vi "Create DiffIO Command.vi"(8 "error in (no error)":errorcluster, 11 "Section Ptr":T5 format="%.0x") -> (0 "error out":errorcluster, 3 "Parent Ref out":T5 format="%.0x")   [LabVIEW 2016, in "DCM System Explorer.lvlib"]
uses:
  DCM System Explorer.lvlib
  <vilib>/NI Veristand/Custom Device API/Custom Device Item Ref.ctl
  <vilib>/Powertrain Controls/Device Drivers/DCM/Diff IO/RT/Setup.ctl
  <vilib>/Powertrain Controls/Device Drivers/DCM/Diff IO/FPGA/Mode.ctl
  <vilib>/Powertrain Controls/Device Drivers/DCM/Diff IO/RT/Angle Control.ctl
  <vilib>/Powertrain Controls/Device Drivers/DCM/Diff IO/RT/Results.ctl
  <vilib>/NI Veristand/Custom Device API/Custom Device Channel Type.ctl
  Shared/DCM Constants and GUIDs.vi
  Shared/DCM Properties.vi
  <vilib>/NI VeriStand/Custom Device API/Custom Device API.lvlib
  DCM Shared.lvlib
  <vilib>/Powertrain Controls/Device Drivers/DCM/Diff IO/RT/DCM - RT - Diff IO.lvlib
  <vilib>/Powertrain Controls/Device Drivers/DCM/Diff IO/FPGA/DCM - FPGA - Diff IO.lvlib
panel:
  in  "Results":T1[](array[typedef]) {"Duty Cycle [%]" format="%#_3g"; "Frequency [Hz]" format="%#_3p"}
  in  "Setup":T2[](array[typedef])=[{"Mode"=enum."Off", "Capture Start [DBTDC]"=0.0, "Capture End [DBTDC]"=0.0, "Invert"=FALSE, "Frequency [Hz]"=0.0, "Duty Cycle [%]"=0.0, "TDC Offset [CAD]"=0.0, "Window Start [DBTDC]"=0.0, "Window End [DBTDC]"=0.0, "Angles"=[{"Enable"=FALSE, "Location [DBTDC]"=0.0, "Duration [s]"=0.0}, {"Enable"=FALSE, "Location [DBTDC]"=0.0, "Duration [s]"=0.0}, {"Enable"=FALSE, "Location [DBTDC]"=0.0, "Duration [s]"=0.0}, {"Enable"=FALSE, "Location [DBTDC]"=0.0, "Duration [s]"=0.0}], "Skip Fire"=FALSE, "Skip Fire Index"=0}, {"Mode"=enum."Off", "Capture Start [DBTDC]"=0.0, "Capture End [DBTDC]"=0.0, "Invert"=FALSE, "Frequency [Hz]"=0.0, "Duty Cycle [%]"=0.0, "TDC Offset [CAD]"=0.0, "Window Start [DBTDC]"=0.0, "Window End [DBTDC]"=0.0, "Angles"=[{"Enable"=FALSE, "Location [DBTDC]"=0.0, "Duration [s]"=0.0}, {"Enable"=FALSE, "Location [DBTDC]"=0.0, "Duration [s]"=0.0}, {"Enable"=FALSE, "Location [DBTDC]"=0.0, "Duration [s]"=0.0}, {"Enable"=FALSE, "Location [DBTDC]"=0.0, "Duration [s]"=0.0}], "Skip Fire"=FALSE, "Skip Fire Index"=0}, {"Mode"=enum."Off", "Capture Start [DBTDC]"=0.0, "Capture End [DBTDC]"=0.0, "Invert"=FALSE, "Frequency [Hz]"=0.0, "Duty Cycle [%]"=0.0, "TDC Offset [CAD]"=0.0, "Window Start [DBTDC]"=0.0, "Window End [DBTDC]"=0.0, "Angles"=[{"Enable"=FALSE, "Location [DBTDC]"=0.0, "Duration [s]"=0.0}, {"Enable"=FALSE, "Location [DBTDC]"=0.0, "Duration [s]"=0.0}, {"Enable"=FALSE, "Location [DBTDC]"=0.0, "Duration [s]"=0.0}, {"Enable"=FALSE, "Location [DBTDC]"=0.0, "Duration [s]"=0.0}], "Skip Fire"=FALSE, "Skip Fire Index"=0}, {"Mode"=enum."Off", "Capture Start [DBTDC]"=0.0, "Capture End [DBTDC]"=0.0, "Invert"=FALSE, "Frequency [Hz]"=0.0, "Duty Cycle [%]"=0.0, "TDC Offset [CAD]"=0.0, "Window Start [DBTDC]"=0.0, "Window End [DBTDC]"=0.0, "Angles"=[{"Enable"=FALSE, "Location [DBTDC]"=0.0, "Duration [s]"=0.0}, {"Enable"=FALSE, "Location [DBTDC]"=0.0, "Duration [s]"=0.0}, {"Enable"=FALSE, "Location [DBTDC]"=0.0, "Duration [s]"=0.0}, {"Enable"=FALSE, "Location [DBTDC]"=0.0, "Duration [s]"=0.0}], "Skip Fire"=FALSE, "Skip Fire Index"=0}, {"Mode"=enum."Off", "Capture Start [DBTDC]"=0.0, "Capture End [DBTDC]"=0.0, "Invert"=FALSE, "Frequency [Hz]"=0.0, "Duty Cycle [%]"=0.0, "TDC Offset [CAD]"=0.0, "Window Start [DBTDC]"=0.0, "Window End [DBTDC]"=0.0, "Angles"=[{"Enable"=FALSE, "Location [DBTDC]"=0.0, "Duration [s]"=0.0}, {"Enable"=FALSE, "Location [DBTDC]"=0.0, "Duration [s]"=0.0}, {"Enable"=FALSE, "Location [DBTDC]"=0.0, "Duration [s]"=0.0}, {"Enable"=FALSE, "Location [DBTDC]"=0.0, "Duration [s]"=0.0}], "Skip Fire"=FALSE, "Skip Fire Index"=0}, {"Mode"=enum."Off", "Capture Start [DBTDC]"=0.0, "Capture End [DBTDC]"=0.0, "Invert"=FALSE, "Frequency [Hz]"=0.0, "Duty Cycle [%]"=0.0, "TDC Offset [CAD]"=0.0, "Window Start [DBTDC]"=0.0, "Window End [DBTDC]"=0.0, "Angles"=[{"Enable"=FALSE, "Location [DBTDC]"=0.0, "Duration [s]"=0.0}, {"Enable"=FALSE, "Location [DBTDC]"=0.0, "Duration [s]"=0.0}, {"Enable"=FALSE, "Location [DBTDC]"=0.0, "Duration [s]"=0.0}, {"Enable"=FALSE, "Location [DBTDC]"=0.0, "Duration [s]"=0.0}], "Skip Fire"=FALSE, "Skip Fire Index"=0}, {"Mode"=enum."Off", "Capture Start [DBTDC]"=0.0, "Capture End [DBTDC]"=0.0, "Invert"=FALSE, "Frequency [Hz]"=0.0, "Duty Cycle [%]"=0.0, "TDC Offset [CAD]"=0.0, "Window Start [DBTDC]"=0.0, "Window End [DBTDC]"=0.0, "Angles"=[{"Enable"=FALSE, "Location [DBTDC]"=0.0, "Duration [s]"=0.0}, {"Enable"=FALSE, "Location [DBTDC]"=0.0, "Duration [s]"=0.0}, {"Enable"=FALSE, "Location [DBTDC]"=0.0, "Duration [s]"=0.0}, {"Enable"=FALSE, "Location [DBTDC]"=0.0, "Duration [s]"=0.0}], "Skip Fire"=FALSE, "Skip Fire Index"=0}, {"Mode"=enum."Off", "Capture Start [DBTDC]"=0.0, "Capture End [DBTDC]"=0.0, "Invert"=FALSE, "Frequency [Hz]"=0.0, "Duty Cycle [%]"=0.0, "TDC Offset [CAD]"=0.0, "Window Start [DBTDC]"=0.0, "Window End [DBTDC]"=0.0, "Angles"=[{"Enable"=FALSE, "Location [DBTDC]"=0.0, "Duration [s]"=0.0}, {"Enable"=FALSE, "Location [DBTDC]"=0.0, "Duration [s]"=0.0}, {"Enable"=FALSE, "Location [DBTDC]"=0.0, "Duration [s]"=0.0}, {"Enable"=FALSE, "Location [DBTDC]"=0.0, "Duration [s]"=0.0}], "Skip Fire"=FALSE, "Skip Fire Index"=0}] {"Skip Fire Index" max=7; "Angles"."Duration [s]" format="%#_3p"; "Frequency [Hz]" format="%#_3p"}
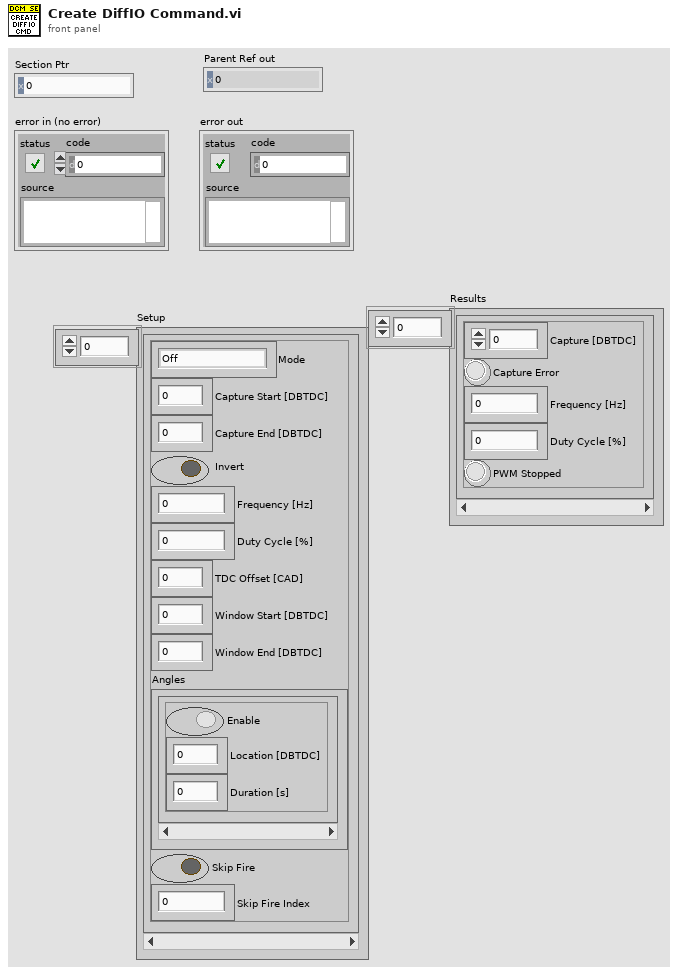
[diagram p1: front panel]
types:
  T1 = typedef "DCM - RT - Diff IO.lvlib/Results.ctl" = cluster{"Capture [DBTDC]":sgl, "Capture Error":bool, "Frequency [Hz]":sgl, "Duty Cycle [%]":sgl, "PWM Stopped":bool}
  T2 = typedef "DCM - RT - Diff IO.lvlib/Setup.ctl" = cluster{"Mode":T3, "Capture Start [DBTDC]":sgl, "Capture End [DBTDC]":sgl, "Invert":bool, "Frequency [Hz]":sgl, "Duty Cycle [%]":sgl, "TDC Offset [CAD]":sgl, "Window Start [DBTDC]":sgl, "Window End [DBTDC]":sgl, "Angles":T4[], "Skip Fire":bool, "Skip Fire Index":u8}
  T3 = typedef "DCM - FPGA - Diff IO.lvlib/Mode.ctl" = enum8{"Off", "Input", "Pulse Width Modulation", "Engine Position Tracking", "Serial Out 1", "Serial Out 2", "EPTx Sync"}
  T4 = typedef "DCM - RT - Diff IO.lvlib/Angle Control.ctl" = cluster{"Enable":bool, "Location [DBTDC]":sgl, "Duration [s]":sgl}
  T5 = typedef "Custom Device API.lvlib/Custom Device Item Ref.ctl" = u64
  T6 = typedef "Custom Device API.lvlib/Custom Device Channel Type.ctl" = enum16{"Input", "Output"}
  T7 = typedef "DCM Shared.lvlib/Channel.ctl" = cluster{"Name":string, "Units":string, "Default":dbl, "Description":string}
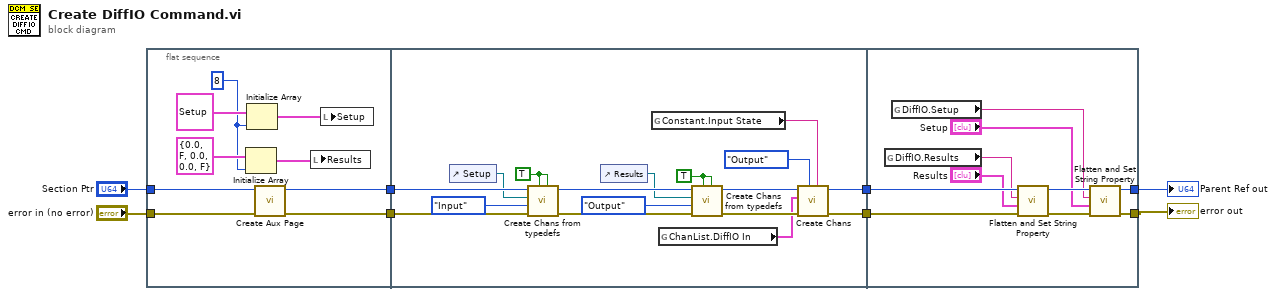
[diagram p0: block diagram]
diagram:
  n1 = flat-sequence {
    tunnel: [w11] -> w7
    tunnel: [w9] -> w8
    tunnel: "error in (no error)" -> [w10]
    tunnel: "Section Ptr" -> [w17]
    tunnel: [w20] -> w6
    tunnel: [w24] -> w5
    tunnel: w8 -> [w32]
    tunnel: w7 -> [w33]
    tunnel: [w39] -> w2
    tunnel: w6 -> [w43]
    tunnel: w5 -> [w44]
    tunnel: [w35] -> w1
    frame #0 {
      w12 = 8 ("dimension size")
      n2 = Initialize Array(T1 {"Capture [DBTDC]"=0.0, "Capture Error"=FALSE, "Frequency [Hz]"=0.0, "Duty Cycle [%]"=0.0, "PWM Stopped"=FALSE} ("Diff I/O Result"), w12) -> (w15:T1[])
      n3 = Initialize Array(T2 {"Mode"=enum."Off", "Capture Start [DBTDC]"=0.0, "Capture End [DBTDC]"=0.0, "Invert"=FALSE, "Frequency [Hz]"=0.0, "Duty Cycle [%]"=0.0, "TDC Offset [CAD]"=0.0, "Window Start [DBTDC]"=0.0, "Window End [DBTDC]"=0.0, "Angles"=[{"Enable"=FALSE, "Location [DBTDC]"=0.0, "Duration [s]"=0.0}, {"Enable"=FALSE, "Location [DBTDC]"=0.0, "Duration [s]"=0.0}, {"Enable"=FALSE, "Location [DBTDC]"=0.0, "Duration [s]"=0.0}, {"Enable"=FALSE, "Location [DBTDC]"=0.0, "Duration [s]"=0.0}], "Skip Fire"=FALSE, "Skip Fire Index"=0} ("PWM Control 2"), w12) -> (w13:T2[])
      n4 = call "Create Aux Page.vi"("error in (no error)"=w10, "Section Ptr"=w17) -> ("error out"=w9:errorcluster, "Parent Ref out"=w11:T5)  [unwired: 8 in]
      n5 = local write "Results"(w15) -> ()
      n6 = local write "Setup"(w13) -> ()
    }
    frame #1 {
      w28 = TRUE ("Prevent overwrite? (F)")
      w27 = TRUE ("Prevent overwrite? (F)")
      n7 = control-ref of="Setup"() -> (w19:refnum<vi>)
      n8 = call "Create Chans from typedefs.vi"("Default from text? (F)"=w27, "Prevent overwrite? (F)"=w27, "error in"=w32, "Type"=Custom_Device_Channel_Type."Input", "Ctl Ref"=w19, "Section Ref in"=w33) -> ("error out"=w31:errorcluster, "Section Ref out"=w30:T5)  [unwired: 3 in, 1 out]
      n9 = control-ref of="Results"() -> (w18:refnum<vi>)
      n10 = global read "DCM Constants and GUIDs.vi" "Constant.Input State"() -> (w21:string)
      n11 = global read "DCM Constants and GUIDs.vi" "ChanList.DiffIO In"() -> (w23:T7[])
      n12 = call "Create Chans from typedefs.vi"("Default from text? (F)"=w28, "Prevent overwrite? (F)"=w28, "error in"=w31, "Type"=Custom_Device_Channel_Type."Output", "Ctl Ref"=w18, "Section Ref in"=w30) -> ("error out"=w25:errorcluster, "Section Ref out"=w26:T5)  [unwired: 3 in, 1 out]
      n13 = call "Create Chans.vi"("New Section Name (none)"=w21, "Type"=Custom_Device_Channel_Type."Output", "error in (no error)"=w25, "Channels"=w23, "Section Ptr"=w26) -> ("error out"=w24:errorcluster, "Section Ptr dup"=w20:T5)  [unwired: 3 in, 2 out]
    }
    frame #2 {
      n14 = global read "DCM Properties.vi" "DiffIO.Results"() -> (w42:string)
      n15 = global read "DCM Properties.vi" "DiffIO.Setup"() -> (w37:string)
      n16 = call "Flatten and Set String Property.vi"("error in (no error)"=w44, "Value"="Results", "Property Name"=w42, "Section Ref in"=w43) -> ("error out"=w40:errorcluster, "Section Ref out"=w38:T5)  [unwired: 6 in]
      n17 = call "Flatten and Set String Property.vi"("error in (no error)"=w40, "Value"="Setup", "Property Name"=w37, "Section Ref in"=w38) -> ("error out"=w39:errorcluster, "Section Ref out"=w35:T5)  [unwired: 6 in]
    }
  }
  "Parent Ref out" <- w1
  "error out" <- w2
